vi "Parse Object Properties.vi"(11 "JSON String":string) -> (0 "Empty Container?":bool, 1 "Values":string[](array[string]), 2 "Item Types":T1[](array[typedef]), 3 "Keys":string[](array[string]))   [LabVIEW 2020, in "JSON.lvlib"]
uses:
  JSON.lvlib
  JSON Item Type.ctl
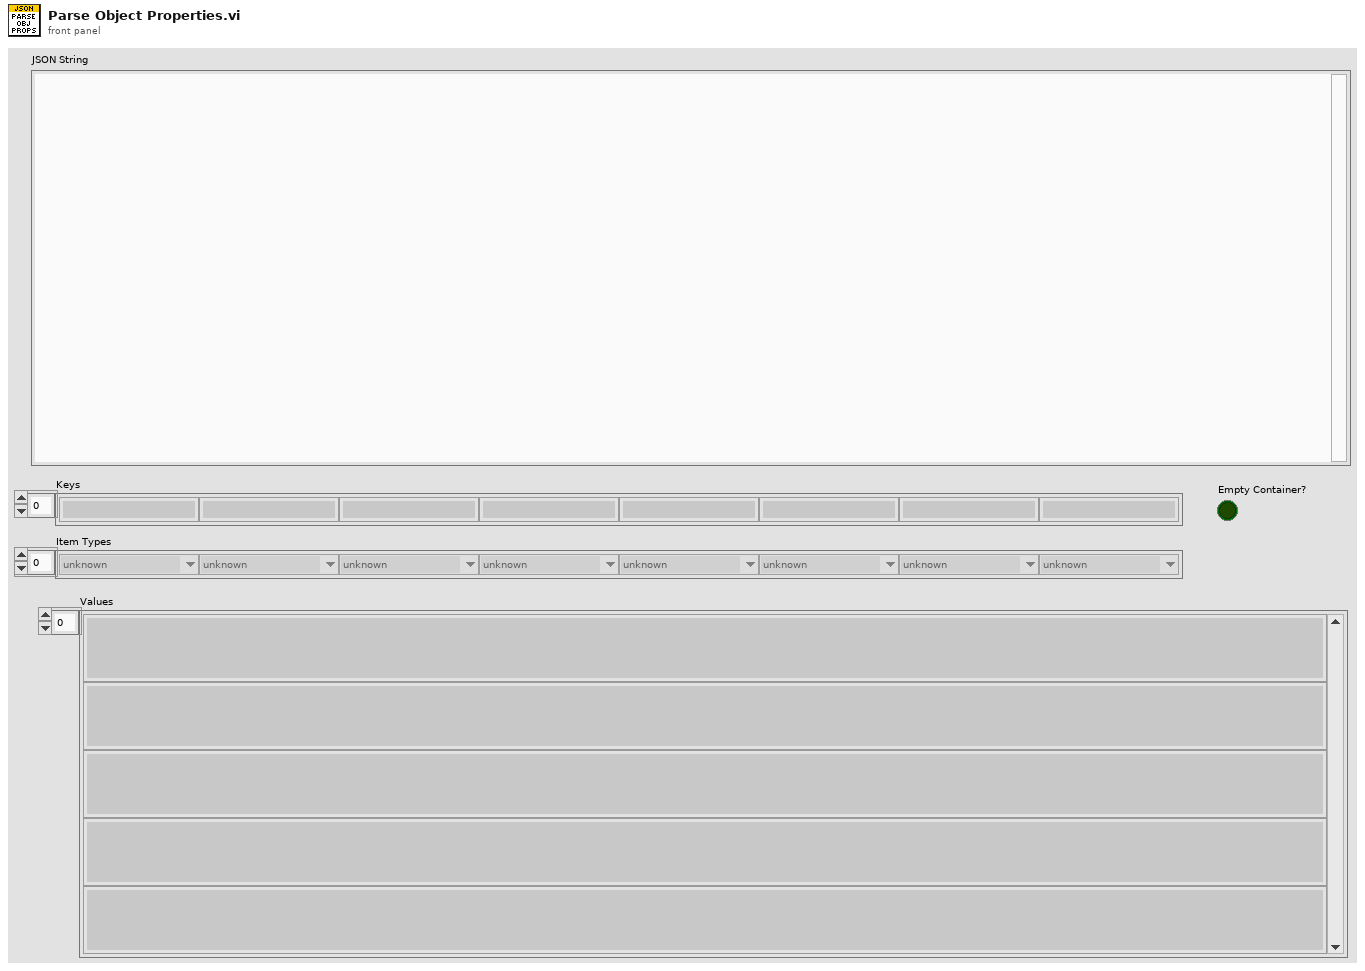
[diagram p1: front panel]
types:
  T1 = typedef "JSON.lvlib/JSON Item Type.ctl" = enum16{"unknown", "null", "Array", "Object", "String", "Number", "Boolean"}
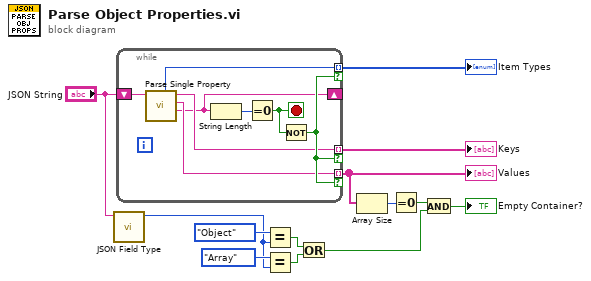
[diagram p0: block diagram]
diagram:
  n1 = call "JSON Field Type.vi"("JSON String"="JSON String") -> ("JSON Item Type"=w4:T1)  [unwired: 10 in]
  n2 = while {
    shift-right: [w14] -> _
    shift-left: "JSON String" -> [w18]
    tunnel: [w16] -> w13 mode=indexing if=w19
    tunnel: [w15] -> w9 mode=indexing if=w19
    tunnel: [w17] -> w12 mode=indexing if=w19
    stop <- w20 stop-if-true
    n3 = call "Parse Single Property.vi"("String In"=w18) -> ("Remaining"=w14:string, "Value"=w15:string, "Key"=w16:string, "JSON Item Type"=w17:T1)  [unwired: 7 in]
    n4 = String Length(string=w14) -> (length=w21:i32)
    n5 = Equal To 0?(x=w21) -> (x = 0?=w20:bool)
    n6 = Not(x=w20) -> (.not. x?=w19:bool)
  }
  "Keys" <- w13
  "Values" <- w9
  "Item Types" <- w12
  n7 = Equal?(x=JSON_Item_Type."Object", y=w4) -> (x = y?=w3:bool)
  n8 = Equal?(x=JSON_Item_Type."Array", y=w4) -> (x = y?=w2:bool)
  n9 = Or(x=w3, y=w2) -> (x .or. y?=w1:bool)
  n10 = Array Size(array=w9) -> (size(s)=w8:i32)
  n11 = Equal To 0?(x=w8) -> (x = 0?=w7:bool)
  n12 = And(x=w7, y=w1) -> (x .and. y?=→"Empty Container?":bool)
